vi "otherInit.vi"() -> ()   [LabVIEW 2018]
panel:
  in  "扫描模式":string[](array[string])
  in  "测量距离":dbl=150.0
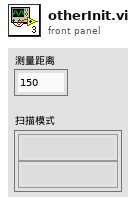
[diagram p1: front panel]
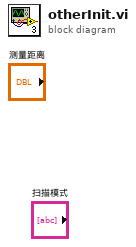
[diagram p0: block diagram]
diagram:
